vi "station_keeping_details.vi"(8 "error in (no error)":errorcluster, 11 "Mission in":refnum<class "Mission.lvclass">) -> (0 "error out":errorcluster, 1 "Buoy SE":T1 {"North" format="%#_10f"; "East" format="%#_8f"}, 2 "Buoy NE":T1 {"North" format="%#_10f"; "East" format="%#_8f"}, 3 "Mission out":refnum<class "Mission.lvclass">, 4 "Buoy SW":T1 {"North" format="%#_10f"; "East" format="%#_8f"}, 5 "Buoy NW":T1 {"North" format="%#_10f"; "East" format="%#_8f"}, 6 "Station Mdpt":T1 {"North" format="%#_10f"; "East" format="%#_8f"})   [LabVIEW 2011, in "Mission.lvclass"]
uses:
  Mission.lvclass
  2 Typedefs/UTM Location.ctl
  Mission.lvclass/Mission.ctl
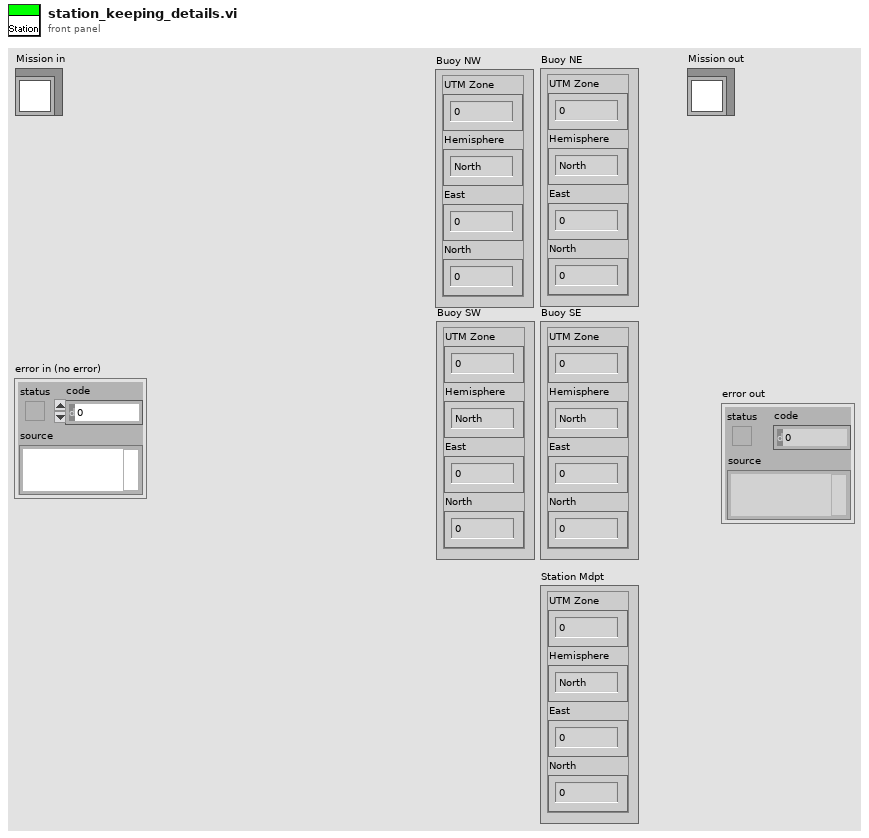
[diagram p1: front panel]
types:
  T1 = typedef "UTM Location.ctl" = cluster{"UTM Zone":dbl, "Hemisphere":enum16{"North", "South"}, "East":dbl, "North":dbl}
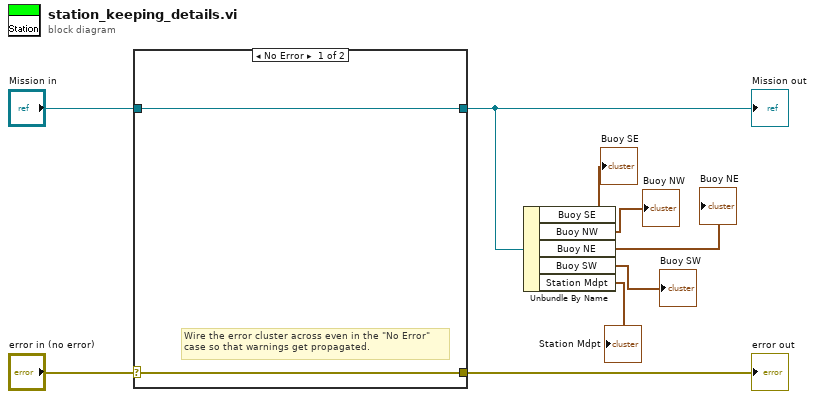
[diagram p0: block diagram]
diagram:
  n1 = case shown="No Error" "error in (no error)" {
    selector: "error in (no error)" -> [w10 w13]
    tunnel: [w10 w13] -> w8
    tunnel: [w11 w12] -> w6
    tunnel: "Mission in" -> [w11 w12]
    frame No Error {
      # "Wire the error cluster across even in the \"No Error\"\ncase so that warnings get propagated."
    }
    frame Error {
    }
  }
  "error out" <- w8
  "Mission out" <- w6
  n2 = Unbundle By Name(w6) -> ("Buoy SE"=→"Buoy SE":T1, "Buoy NW"=→"Buoy NW":T1, "Buoy NE"=→"Buoy NE":T1, "Buoy SW"=→"Buoy SW":T1, "Station Mdpt"=→"Station Mdpt":T1)
